vi "SDT_Generate_bhfile_header.vi"(4 "setup_length":i32, 5 "no_of_data_blocks":u32, 6 "adc_re[dig]":u32, 7 "info_length":i32, 9 "ImageSize":u32, 10 "NoOfRoutingChannel":i32, 11 "BHModuleType":T2 format="x%x" items=["SPC-130"=32, "SPC-600"=33, "SPC-630"=34, "SPC-700"=35, "SPC-730"=36, "SPC-830"=37, "SPC-140"=38, "SPC-930"=39, "SPC-150"=40, "DPC-230"=41, "SPC-130EM"=42, "SPC-160"=43, "SPC-150N"=46, "PMS-800"=51, "SPC-150NX"=128, "SPC-160X"=129, "SPC-160PCIE"=130, "SPC-130EMN"=131, "SPC-180N"=132, "SPC-180NX"=133, "SPC-180NXX"=134, "SPC-180N-USB"=135, "SPC-130IN"=136, "SPC-130INX"=137, "SPC-130INXX"=138, "SPC-QC-104"=139, "Simulation"=-1]) -> (2 "data_block_offs":i32, 3 "bhfile_header":T1)   [LabVIEW 2017]
doc: "This VI is a SubVI to SDT_WriteFile.vi. It populates the bhfile_header cluster ready to be written to file. \nFor a description of the *.sdt file format see: SPC_data_file_structure.h\n\ninfo@becker-hickl.com"
uses:
  SPC_Wrappers/SPC_Controls/BHModuleType.ctl
  SPC_Wrappers/SPC_Controls/bhfile_header.ctl
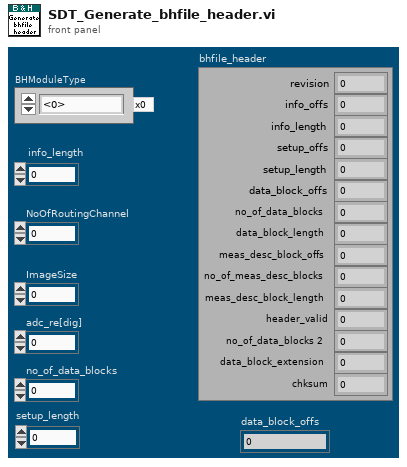
[diagram p1: front panel]
types:
  T1 = typedef "bhfile_header.ctl" = cluster{"revision":i16, "info_offs":i32, "info_length":i16, "setup_offs":i32, "setup_length":u16, "data_block_offs":i32, "no_of_data_blocks":i16, "data_block_length":u32, "meas_desc_block_offs":i32, "no_of_meas_desc_blocks":i16, "meas_desc_block_length":i16, "header_valid":u16, "no_of_data_blocks 2":u32, "data_block_extension":u16, "chksum":u16}
  T2 = typedef "BHModuleType.ctl" = i16
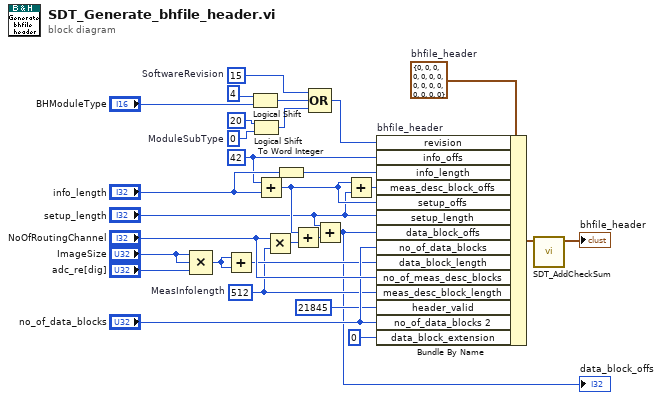
[diagram p0: block diagram]
diagram:
  w6 = 42 ("Info Offset")
  w7 = T1 {"revision"=0, "info_offs"=0, "info_length"=0, "setup_offs"=0, "setup_length"=0, "data_block_offs"=0, "no_of_data_blocks"=0, "data_block_length"=0, "meas_desc_block_offs"=0, "no_of_meas_desc_blocks"=0, "meas_desc_block_length"=0, "header_valid"=0, "no_of_data_blocks 2"=0, "data_block_extension"=0, "chksum"=0}  # bhfile_header
  w20 = 512  # MeasInfolength
  w19 = i16 0  # ModuleSubType
  w14 = i16 15  # SoftwareRevision
  n1 = Compound Arithmetic op=MULTIPLY("ImageSize", "ImageSize", "adc_re[dig]") -> (w22:u32)
  n2 = Add(x=w22, y=w22) -> (x+y=w21:u32)
  n3 = Logical Shift(y=i16 4, x="BHModuleType") -> (x << y=w15:T2)
  n4 = Logical Shift(y=i16 20, x=w19) -> (x << y=w18:i16)
  n5 = Add(x=w6, y="info_length") -> (x+y=w3:i32)
  n6 = Multiply(x="NoOfRoutingChannel", y=w20) -> (x*y=w26:i32)
  n7 = To Word Integer(number="info_length") -> (16bit integer=w5:i16)
  n8 = Add(x=w3, y=w26) -> (x+y=w25:i32)
  n9 = Compound Arithmetic op=OR(w14, w15, w18) -> (w16:T2)
  n10 = Add(x="setup_length", y=w25) -> (x+y=w2:i32)
  "data_block_offs" <- w2
  n11 = Add(x=w3, y="setup_length") -> (x+y=w4:i32)
  n12 = Bundle By Name "bhfile_header"(cluster=w7, "revision"=w16, "info_offs"=w6, "info_length"=w5, "meas_desc_block_offs"=w4, "setup_offs"=w3, "setup_length"="setup_length", "data_block_offs"=w2, "no_of_data_blocks"="no_of_data_blocks", "data_block_length"=w21, "no_of_meas_desc_blocks"="NoOfRoutingChannel", "meas_desc_block_length"=w20, "header_valid"=u16 21845, "no_of_data_blocks 2"="no_of_data_blocks", "data_block_extension"=u16 0) -> (w11:T1)
  n13 = call "SDT_AddCheckSum.vi"("bhfile_header"=w11) -> ("HeaderWithChkSum"=→"bhfile_header":T1)  [unwired: 9 in, 1 out]
